vi "p1230 read port.vi"(8 "error in (no error)":errorcluster, 10 "pData":u32, 11 "board_id":u32) -> (0 "error out":errorcluster, 2 "pData out":u32, 3 "function return":u32)   [LabVIEW 2014]
doc: "unsigned int __stdcall p1230_read_port(unsigned int board_id, unsigned int* pData);"
uses:
  PCI1230UTIL.dll
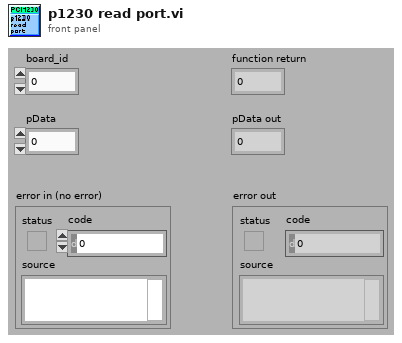
[diagram p1: front panel]
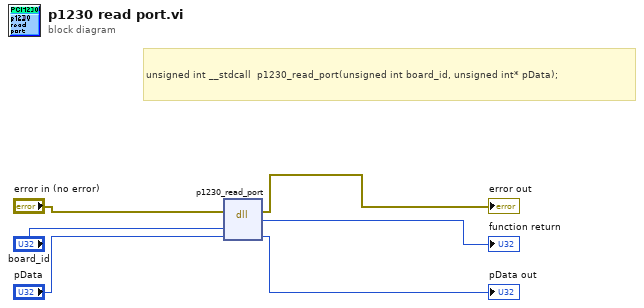
[diagram p0: block diagram]
diagram:
  # "unsigned int __stdcall  p1230_read_port(unsigned int board_id, unsigned int* pData);"
  n1 = dll-call lib="C:/Users/AICTER/Desktop/PCI-1230/PCI1230_VIs/PCI1230UTIL.*" fn="p1230_read_port"(error in="error in (no error)", "board_id"="board_id", "pData"="pData") -> (error out=→"error out":errorcluster, →"function return":u32, "pData"=→"pData out":u32)  [unwired: 3 in, 1 out]
